vi "Brace_Init.vi"(8 "error in (no error)":errorcluster, 10 "Serial Settings":T1, 11 "VISA Refnum in":refnum<visa-resource-name>) -> (1 "Initialised":bool, 2 "Connected":bool, 5 "Data Out":string)   [LabVIEW 2018]
panel:
  out "error out 2":errorcluster
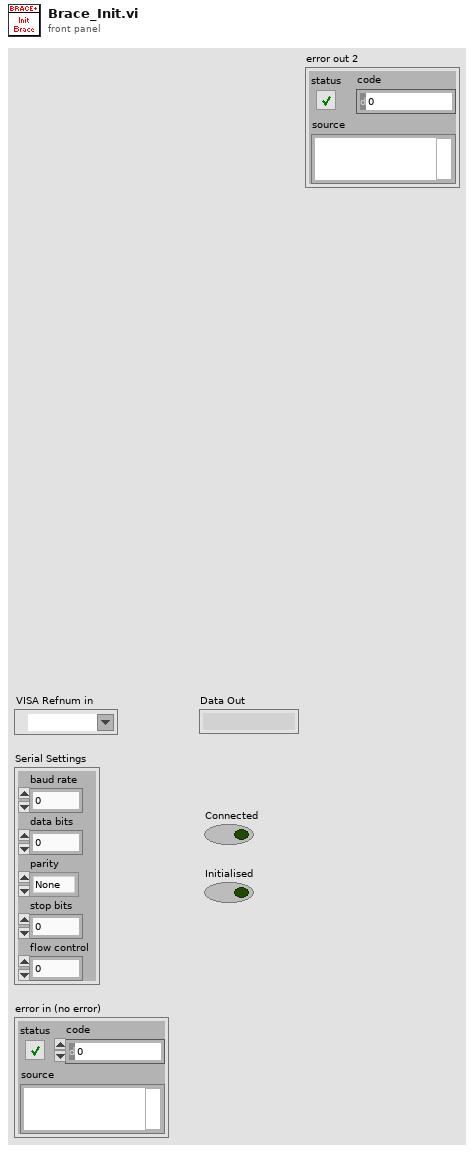
[diagram p1: front panel]
types:
  T1 = cluster{"baud rate":u32, "data bits":u16, "parity":enum16{"None", "Odd", "Even", "Mark", "Space"}, "stop bits":u16, "flow control":u16}
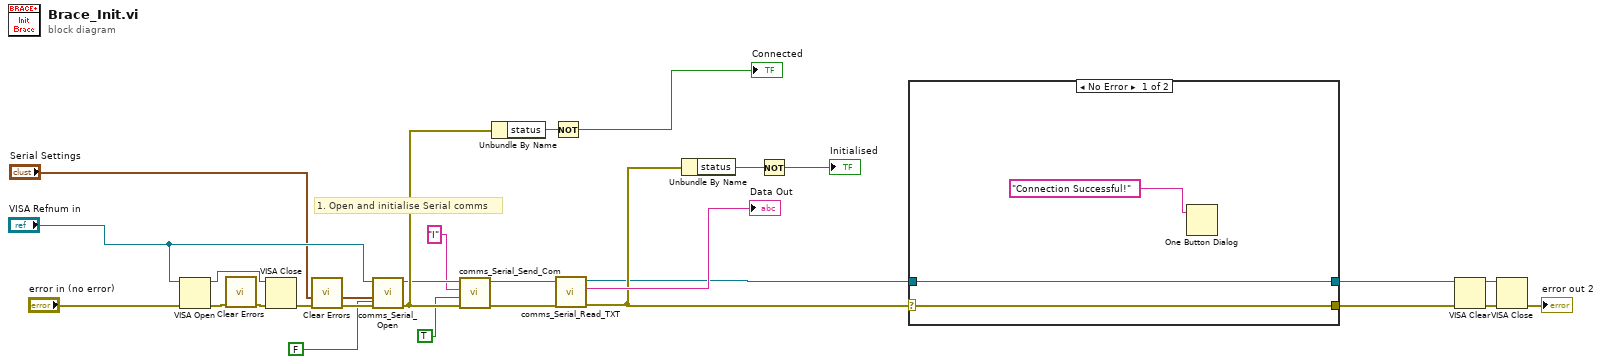
[diagram p0: block diagram]
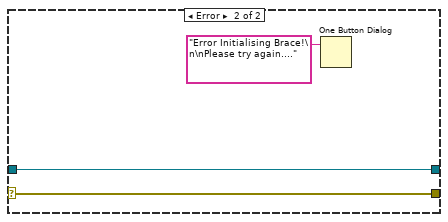
[diagram p2: hidden frame]
diagram:
  # "1. Open and initialise Serial comms"
  n1 = VISA Open(error in (no error)="error in (no error)", VISA resource name="VISA Refnum in") -> (VISA resource name=w21:refnum<visa-resource-name>, error out=w22:errorcluster)  [unwired: 3 in]
  n2 = call <vilib>:"Clear Errors.vi"("error in (no error)"=w22) -> ("error out"=w23:errorcluster)  [unwired: 5 in, 1 out]
  n3 = VISA Close(VISA resource name=w21, error in (no error)=w23) -> (error out=w24:errorcluster)
  n4 = call <vilib>:"Clear Errors.vi"("error in (no error)"=w24) -> ("error out"=w25:errorcluster)  [unwired: 5 in, 1 out]
  n5 = call "comms_Serial_Open.vi"("Send Init Comm?"=FALSE, "error in (no error)"=w25, "Serial Settings in"="Serial Settings", "VISA Refnum in"="VISA Refnum in") -> ("error out"=w27:errorcluster, "VISA Refnum out"=w12:refnum<visa-resource-name>)  [unwired: 5 in, 1 out]
  n6 = call "comms_Serial_Send_Com.vi"("error in"=w27, "Buffer Clear?"=TRUE, "Command"="I", "VISA resource in"=w12) -> ("error out"=w26:errorcluster, "VISA resource Out"=w14:refnum<visa-resource-name>)  [unwired: 5 in, 1 out]
  n7 = Unbundle By Name(w27) -> ("status"=w16:bool)
  n8 = Not(x=w16) -> (.not. x?=→"Connected":bool)
  n9 = call "comms_Serial_Read_TXT.vi"("error in"=w26, "VISA resource in"=w14) -> ("error out"=w3:errorcluster, "Data Out"=→"Data Out":string, "VISA resource Out"=w2:refnum<visa-resource-name>)  [unwired: 6 in, 1 out]
  n10 = Unbundle By Name(w3) -> ("status"=w17:bool)
  n11 = Not(x=w17) -> (.not. x?=→"Initialised":bool)
  n12 = case shown="No Error" w3 {
    selector: w3 -> [w29 w32]
    tunnel: [w30 w33] -> w6
    tunnel: [w29 w32] -> w5
    tunnel: w2 -> [w30 w33]
    frame No Error {
      n13 = One Button Dialog(message="Connection Successful!") -> ()  [unwired: 1 in, 1 out]
    }
    frame Error {
      n14 = One Button Dialog(message="Error Initialising Brace!\n\nPlease try again....") -> ()  [unwired: 1 in, 1 out]
    }
  }
  n15 = VISA Clear(VISA resource name=w6, error in (no error)=w5) -> (VISA resource name out=w8:refnum<visa-resource-name>, error out=w7:errorcluster)
  n16 = VISA Close(VISA resource name=w8, error in (no error)=w7) -> (error out=→"error out 2":errorcluster)
